vi "Execute Value Update Policy.vi"(8 "error in (no error)":errorcluster, 9 "Publish Time":timestamp, 10 "New Topic Value":variant, 11 "BasicSubscription In":refnum<class "BasicSubscription.lvclass">) -> (0 "error out":errorcluster, 3 "BasicSubscription Out":refnum<class "BasicSubscription.lvclass">)   [LabVIEW 2017, in "SubscriptionPolicy.lvlib" / "BasicSubscription.lvclass"]
uses:
  BasicSubscription.lvclass
  C:/Git/mva-framework/Source/Framework/IMediator/ISubscriptionPolicy/ISubscriptionPolicy.lvclass
  IMediator/ISubscriptionPolicy/ISubscriptionPolicy.lvclass/ISubscriptionPolicy.ctl
  gpm_packages/@cs/transport/Source/ITransport/Transport Data.vi
  gpm_packages/@cs/transport/Source/ITransport/ITransport.lvclass
  IMediator/ISubscriptionPolicy/ISubscriptionPolicy.lvclass
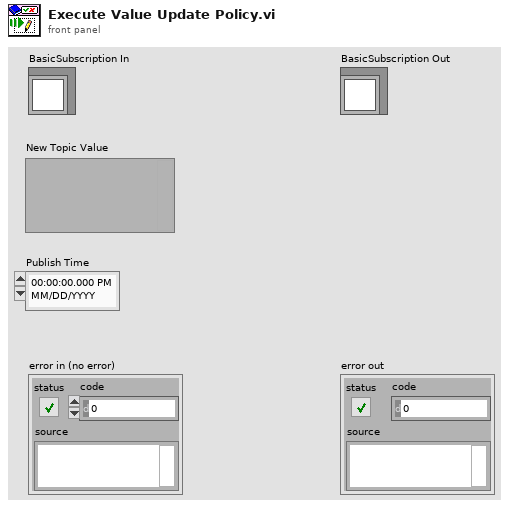
[diagram p1: front panel]
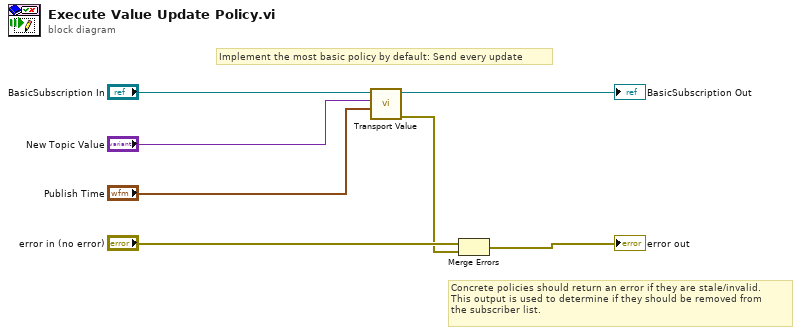
[diagram p0: block diagram]
diagram:
  # "Implement the most basic policy by default: Send every update"
  # "Concrete policies should return an error if they are stale/invalid.\nThis output is used to determine if they should be removed from\nthe subscriber list."
  n1 = call "Transport Value.vi"("Publish Time"="Publish Time", "Value"="New Topic Value", "ISubscriptionPolicy in"="BasicSubscription In") -> ("error out"=w1:errorcluster, "ISubscriptionPolicy out"=→"BasicSubscription Out":refnum<class "BasicSubscription.lvclass">)  [unwired: 7 in]
  n2 = Merge Errors("error in (no error)", w1) -> (→"error out":errorcluster)
